vi "G1.vi"() -> ()   [LabVIEW 2015]
panel:
  in  "2":bool
  in  "1":bool
  in  "Stop Button":bool
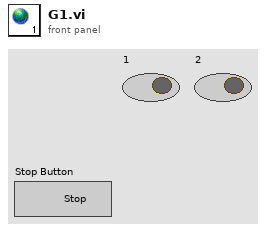
[diagram p1: front panel]
diagram:
